vi "From Scanreader XML String.vi"(11 "xml string":string) -> (0 "Use LCD?":bool, 1 "Reader":T2, 2 "Scanner 2 (second scan axis)":T1=enum."None", 3 "Scanner":T1)   [LabVIEW 2017, in "Scan Driver.lvclass"]
uses:
  Scan Driver.lvclass
  Reader List.ctl
  Scanner List.ctl
panel:
  out "output cluster":T3
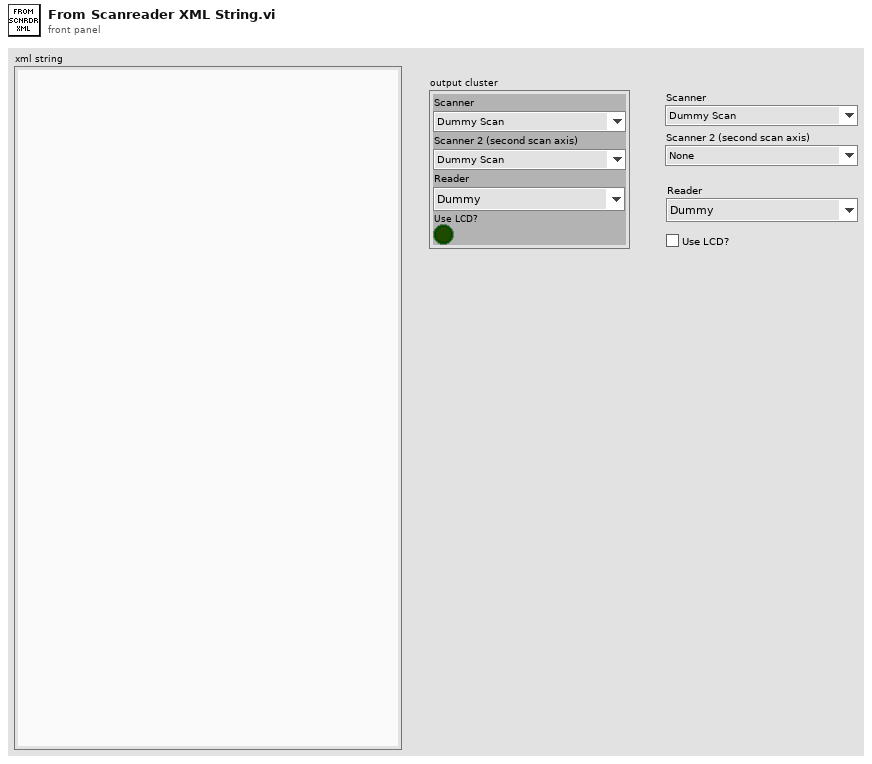
[diagram p1: front panel]
types:
  T1 = typedef "Scan Driver.lvclass/Scanner List.ctl" = enum16{"Dummy Scan", "Analog Output Scan", "Function Gen Scan", "Magna Current Scan", "Magna Voltage Scan", "Magnetic Field Lakeshore", "Magnetic Field Lakeshore Continuous", "Magnetic Field Oxford", "Magnetic Field Oxford Continuous", "Microwave Freq Scan", "Pulse Gen Basic Scan", "Pulse Gen Scan", "Translation Stage Coarse", "Translation Stage Dual", "Translation Stage Fine", "Wavelength ActiveX", "Wavelength Digikröm", "Wavelength PEM and Digikröm", "Wavelength Triax 550", "None"}
  T2 = typedef "Scan Driver.lvclass/Reader List.ctl" = enum16{"Dummy", "Cryostat Temperature", "DAQmx Analog", "Fluke Multimeter", "Keithley Multimeter", "Lockin SR810", "Lockin SR830", "Lockin and Fluke Multimeter", "Photon Counter Reader", "Photon Counter w/ LCD", "Power Meter", "Temperature Control", "Two Lockins"}
  T3 = cluster{"Scanner":T1, "Scanner 2 (second scan axis)":T1, "Reader":T2, "Use LCD?":bool}
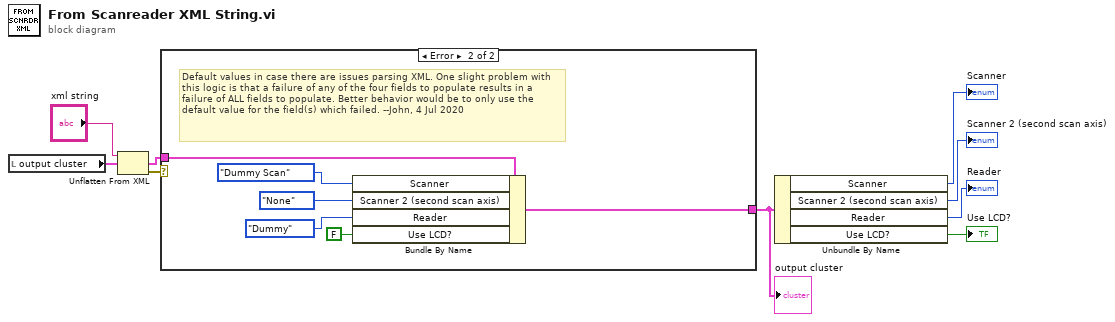
[diagram p0: block diagram]
diagram:
  n1 = local read "output cluster"() -> (w8:T3)
  n2 = Unflatten From XML(xml string="xml string", type=w8) -> (value=w2:T3, error out=w3:errorcluster)  [unwired: 1 in]
  n3 = case shown="Error" w3 {
    tunnel: w2 -> [w10 w16]
    tunnel: [w10 w11] -> w1
    frame No Error {
    }
    frame Error {
      # "Default values in case there are issues parsing XML. One slight problem with this logic is that a failure of any of the four fields to populate results in a failure of ALL fields to populate. Better behavior would be to only use the default value for the field(s) which failed. --John, 4 Jul 2020"
      n4 = Bundle By Name(cluster=w16, "Scanner"=Scanner_List."Dummy Scan", "Scanner 2 (second scan axis)"=Scanner_List."None", "Reader"=Reader_List."Dummy", "Use LCD?"=FALSE) -> (w11:T3)
    }
  }
  "output cluster" <- w1
  n5 = Unbundle By Name(w1) -> ("Scanner"=→"Scanner":T1, "Scanner 2 (second scan axis)"=→"Scanner 2 (second scan axis)":T1, "Reader"=→"Reader":T2, "Use LCD?"=→"Use LCD?":bool)
